vi "TestReset.vi"   [LabVIEW 2016]
uses:
  <vilib>/National Instruments/IoT Education Toolkit Beta/TW API/Thing.lvclass
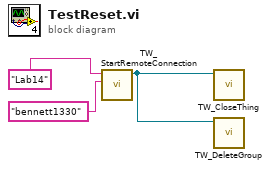
[diagram p0: block diagram]
diagram:
  n1 = call <vilib>:"TW_StartRemoteConnection.vi"("Remote Username"="bennett1330", "Remote ThingName"="Lab14") -> ("Thing Out"=w1:refnum<class "Thing.lvclass">)  [unwired: 8 in, 1 out]
  n2 = call <vilib>:"TW_CloseThing.vi"("Thing In"=w1) -> ()  [unwired: 6 in, 1 out]
  n3 = call <vilib>:"TW_DeleteGroup.vi"("Thing In"=w1) -> ()  [unwired: 10 in, 1 out]
